vi "Read Multi Eval Meas SEM Trace RBW Results.vi"(6 "Resolution BW (30 kHz)":T1 items=["30 kHz", "100 kHz", "1 MHz", "1% of channel BW", "2% of channel BW"], 8 "error in (no error)":errorcluster, 9 "Result Type (Current)":i32(ring) items=["Current"=0, "Average"=1, "Maximum"=4], 10 "Instance (1)":T2=1, 11 "VISA resource name":refnum<visa-resource-name>) -> (0 "error out":errorcluster, 1 "Results":dbl[](array[numeric]) format="%^.3e", 2 "Reliability":i32, 3 "VISA resource name out":refnum<visa-resource-name>)   [LabVIEW 2020, in "Rohde&Schwarz CMWXP NR FR1 Measurement.lvlib"]
doc: "Returns the values of the spectrum emission traces. Separate traces are available for the individual resolution bandwidths (<kHz>). The results of the current, average and maximum traces can be retrieved.\n\nAttributes:\nRSCMWXPNRFR1M_ATTR_READ_MULTI_EVAL_MEAS_SEM_TRACE_RBW_CURRENT_RESULTS\nRSCMWXPNRFR1M_ATTR_READ_MULTI_EVAL_MEAS_SEM_TRACE_RBW_AVERAGE_RESULTS\nRSCMWXPNRFR1M_ATTR_READ_MULTI_EVAL_MEAS_SEM_TRACE_RBW_MAXIMUM_RESULTS\n\nRemote-control commands:\nREAD:NRSub:MEAS<i>:MEValuation:TRACe:SEMask:RBW<kHz>:CURRent?\nREAD:NRSub:MEAS<i>:MEValuation:TRACe:SEMask:RBW<kHz>:AVERage?\nREAD:NRSub:MEAS<i>:MEValuation:TRACe:SEMask:RBW<kHz>:MAXimum?"
uses:
  <instrlib>/Rohde&Schwarz CMWXP NR FR1 Measurement/Rohde&Schwarz CMWXP NR FR1 Measurement.lvlib
  <instrlib>/Rohde&Schwarz CMWXP NR FR1 Measurement/Private/_Instance.ctl
  <instrlib>/Rohde&Schwarz CMWXP NR FR1 Measurement/Private/_Resolution BW.ctl
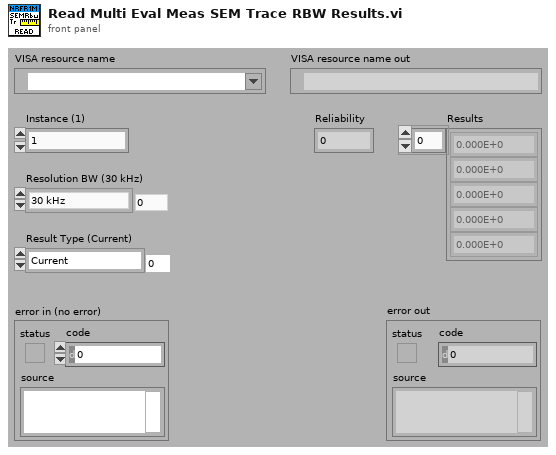
[diagram p1: front panel]
types:
  T1 = typedef "Rohde&Schwarz CMWXP NR FR1 Measurement.lvlib/_Resolution BW.ctl" = i32
  T2 = typedef "Rohde&Schwarz CMWXP NR FR1 Measurement.lvlib/_Instance.ctl" = i32
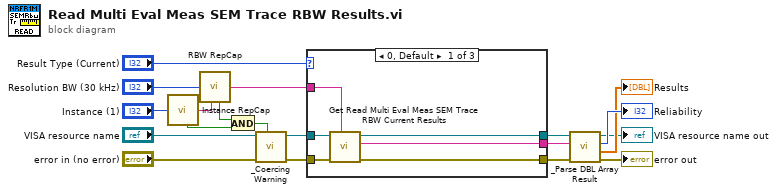
[diagram p0: block diagram]
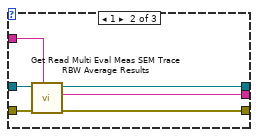
[diagram p2: hidden frame]
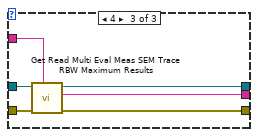
[diagram p3: hidden frame]
diagram:
  n1 = call <instrlib>:"Instance RepCap.vi"("Instance In"="Instance (1)") -> ("In Range?"=w15:bool, "RepCap Identifier Out"=w13:string)  [unwired: 1 in]
  n2 = call <instrlib>:"RBW RepCap.vi"("RBW In"="Resolution BW (30 kHz)", "RepCap String In (\"\")"=w13) -> ("In Range?"=w14:bool, "RepCap Identifier Out"=w12:string)
  n3 = And(x=w14, y=w15) -> (x .and. y?=w16:bool)
  n4 = call <instrlib>:"_Coercing Warning.vi"("In Range?"=w16, "error in (no error)"="error in (no error)", "VISA resource name"="VISA resource name") -> ("error out"=w11:errorcluster, "VISA resource name out"=w10:refnum<visa-resource-name>)  [unwired: 7 in]
  n5 = case shown="0, Default" "Result Type (Current)" {
    tunnel: w12 -> [w25 w31 w37]
    tunnel: w11 -> [w24 w30 w36]
    tunnel: w10 -> [w23 w29 w35]
    tunnel: [w22 w28 w34] -> w5
    tunnel: [w21 w27 w33] -> w6
    tunnel: [w20 w26 w32] -> w7
    frame 0, Default {
      n6 = call "Get Read Multi Eval Meas SEM Trace RBW Current Results"("Repeated Capabilities"=w25, "error in (no error)"=w24, "instrument handle"=w23) -> ("error out"=w20:errorcluster, "Read Multi Eval Meas SEM Trace RBW Current Results"=w21:string, "instrument handle out"=w22:refnum<visa-resource-name>)  [unwired: 6 in]
    }
    frame 1 {
      n7 = call "Get Read Multi Eval Meas SEM Trace RBW Average Results"("Repeated Capabilities"=w31, "error in (no error)"=w30, "instrument handle"=w29) -> ("error out"=w26:errorcluster, "Read Multi Eval Meas SEM Trace RBW Average Results"=w27:string, "instrument handle out"=w28:refnum<visa-resource-name>)  [unwired: 6 in]
    }
    frame 4 {
      n8 = call "Get Read Multi Eval Meas SEM Trace RBW Maximum Results"("Repeated Capabilities"=w37, "error in (no error)"=w36, "instrument handle"=w35) -> ("error out"=w32:errorcluster, "Read Multi Eval Meas SEM Trace RBW Maximum Results"=w33:string, "instrument handle out"=w34:refnum<visa-resource-name>)  [unwired: 6 in]
    }
  }
  n9 = call <instrlib>:"_Parse DBL Array Result.vi"("error in (no error)"=w7, "Input String"=w6, "VISA resource name"=w5) -> ("error out"=→"error out":errorcluster, "Results"=→"Results":dbl[], "Reliability"=→"Reliability":i32, "VISA resource name out"=→"VISA resource name out":refnum<visa-resource-name>)  [unwired: 5 in]
